vi "Read ROI height.vi"(8 "error in (no error)":errorcluster, 11 "Configuration parameters in":refnum<class "CV-Configuration.lvclass">) -> (0 "error out":errorcluster, 2 "ROI height [pixels]":u32=1082 min=1 max=1082 step=1, 3 "Configuration parameters out":refnum<class "CV-Configuration.lvclass">)   [LabVIEW 2013, in "CameraVision.lvlib" / "CV-Configuration.lvclass"]
uses:
  CV-Configuration.lvclass
  CV-Configuration.lvclass/CV-Configuration.ctl
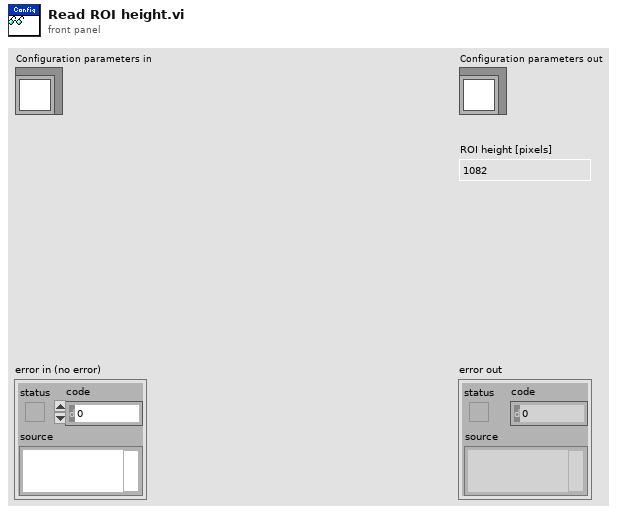
[diagram p1: front panel]
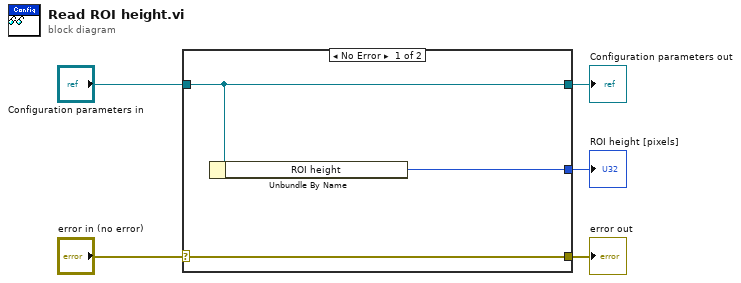
[diagram p0: block diagram]
diagram:
  n1 = case shown="No Error" "error in (no error)" {
    selector: "error in (no error)" -> [w8 w9]
    tunnel: [w8 w9] -> w4
    tunnel: [w7 w10] -> w2
    tunnel: "Configuration parameters in" -> [w7 w10]
    tunnel: [w6 _] -> w1
    frame No Error {
      n2 = Unbundle By Name(w7) -> ("ROI height"=w6:u32)
    }
    frame Error {
    }
  }
  "error out" <- w4
  "Configuration parameters out" <- w2
  "ROI height [pixels]" <- w1
